vi "Load Directional Speed Sensor.vi"(6 "Memory In":refnum<k21>="Directional Gen Memory", 11 "load input.<user name>":T2) -> (0 "done":bool, 2 "load data":T1={"max address"=0.0, "Memory"="Digital Pattern Gen Memory 0"})   [LabVIEW 2013, in "Engine Simulation Toolkit.lvlib" / "Directional Speed.lvlib"]
doc: "Loads data from NI VeriStand into the directional speed sensor memory. <b> This VI should be in an SCTL</b>\n\n<b>load input.<user name></b> - Input for the component. NI VeriStand will set these values. create a control for this input. Replace <user name> with the name you wish this component to display as inside NI VeriStand. Make this name consistent for all controls, indicators, for all VIs of this component.\n<b>memory</b> - Reference to a U16 memory of size 1024. The memory tooth centers. The memory can be set to never arbitrate to save resources.\n\n<b>load data</b> - Information about the loaded memory that should be wired to Directional Speed Sensor.vi\n<b>done</b> - Done loading signal. Wire this to the SCTL stop terminal."
uses:
  Directional Speed.lvlib
  Load Input.ctl
  Load Data.ctl
  <vilib>/rvi/DataTransferAndStorage/Container/Common/niFpgaContainerExecOnDevCompGetState.vi
  <vilib>/rvi/Memory/Memory_Emulation/nirvimemoryFastEmulationFpgaImpl.vi
  <instcachedir>/0/nirvimemoryFastEmulationFpgaImpl_5FBAB50466BC4C939F684F8805638BFC.lvgen/nirvimemoryFastEmulationFpgaImpl_5FBAB50466BC4C939F684F8805638BFC_004.vi
  <vilib>/rvi/DataTransferAndStorage/Container/Common/niFpgaContainerGetUniqueNameForEmu.vi
  <vilib>/rvi/Memory/Memory_Emulation/niFpgaMemoryEmulationCacheClearOnFirstRun.vi
  <vilib>/rvi/Memory/Memory_Emulation/nirvimemoryEmulationManagerCache_MakeExclusive.vi
  <vilib>/rvi/Memory/Memory_Emulation/niFpgaMemoryEmulationValidateCache.vi
  <vilib>/rvi/Memory/Memory_Emulation/nirvimemoryEmulationManagerCache_ReleaseExclusive.vi
  <vilib>/rvi/Memory/Memory_Emulation/nirvimemoryEmulationManagerCache_InsertValue.vi
  <vilib>/Utility/error.llb/Clear Errors.vi
  <vilib>/rvi/Emulation/niFpgaSctlEmulationGetInTimedLoop.vi
  <vilib>/rvi/Memory/Memory_Emulation/nirvimemoryEmulationManagerCache_SetValue.vi
  <vilib>/rvi/Emulation/niFpgaSctlEmulationResourceMgr.vi
  <vilib>/rvi/DataTransferAndStorage/Container/XNode/niFpgaContainer.xnode
  <vilib>/rvi/Memory/Memory_Emulation/niFpgaMemoryEmulationRefIn.vi
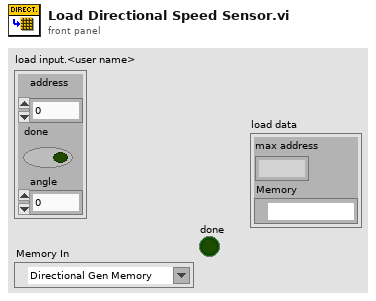
[diagram p1: front panel]
types:
  T1 = typedef "Engine Simulation Toolkit.lvlib/Directional Speed.lvlib/Load Data.ctl" = cluster{"max address":fxp<+,10,10>, "Memory":refnum<k21>}
  T2 = typedef "Engine Simulation Toolkit.lvlib/Directional Speed.lvlib/Load Input.ctl" = cluster{"address":fxp<+,10,10>, "done":bool, "angle":u16}
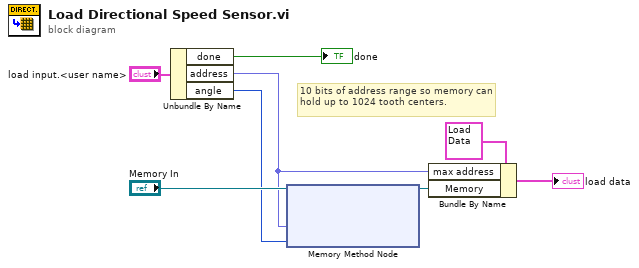
[diagram p0: block diagram]
diagram:
  # "10 bits of address range so memory can hold up to 1024 tooth centers."
  n1 = Unbundle By Name("load input.<user name>") -> ("done"=→"done":bool, "address"=w4:fxp<+,10,10>, "angle"=w3:u16)
  n2 = xnode ("Memory Method Node")("Address"=w4, "Data"=w3, "Memory In"="Memory In") -> ("Memory Out"=w5:refnum<k21>)
  n3 = Bundle By Name(cluster=T1 {"max address"=0.0, "Memory"="Digital Pattern Gen Memory 0"} ("load data"), "max address"=w4, "Memory"=w5) -> (→"load data":T1)
